vi "Filter and Connect Device.vi"() -> ()   [LabVIEW 2022 SP3]
doc: "In this example we will search through available devices to find the first one that has its \nmanufacturer set to 'openDAQ'.Then connect the device into our component tree as a child device."
uses:
  Public/Classes/IInstance/IInstance.lvclass
  Public/Classes/IInstanceBuilder/IInstanceBuilder.lvclass
  Public/Classes/IDevice/IDevice.lvclass
  Public/Classes/IDeviceInfo/IDeviceInfo.lvclass
panel:
  out "connected devices":string[](array[string])
  out "error out":errorcluster
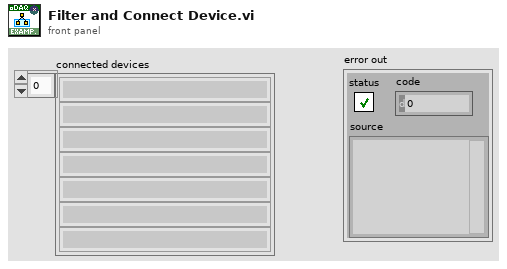
[diagram p1: front panel]
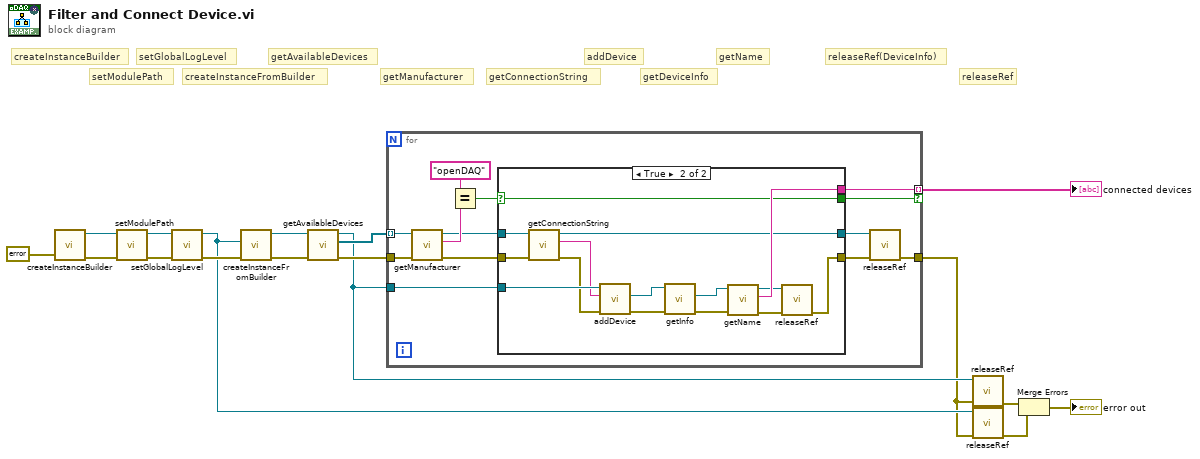
[diagram p0: block diagram]
diagram:
  # "getName"
  # "getDeviceInfo"
  # "addDevice"
  # "getConnectionString"
  # "createInstanceFromBuilder"
  # "releaseRef(DeviceInfo)"
  # "getManufacturer"
  # "releaseRef"
  # "getAvailableDevices"
  # "setGlobalLogLevel"
  # "setModulePath"
  # "createInstanceBuilder"
  n1 = call "createInstanceBuilder.vi"("error in (no error)"=errorcluster {"status"=FALSE, "code"=0, "source"=""}) -> ("error out"=w16:errorcluster, "IInstanceBuilder out"=w15:refnum<class "IInstanceBuilder.lvclass">)  [unwired: 9 in]
  n2 = call "setModulePath.vi"("error in (no error)"=w16, "IInstanceBuilder in"=w15) -> ("error out"=w14:errorcluster, "IInstanceBuilder out"=w13:refnum<class "IInstanceBuilder.lvclass">)  [unwired: 8 in]
  n3 = call "setGlobalLogLevel.vi"("error in (no error)"=w14, "IInstanceBuilder in"=w13) -> ("error out"=w11:errorcluster, "IInstanceBuilder out"=w7:refnum<class "IInstanceBuilder.lvclass">)  [unwired: 8 in]
  n4 = call "createInstanceFromBuilder.vi"("error in (no error)"=w11, "IInstanceBuilder in"=w7) -> ("error out"=w10:errorcluster, "IInstance out"=w9:refnum<class "IInstance.lvclass">)  [unwired: 8 in]
  n5 = call "getAvailableDevices.vi"("error in (no error)"=w10, "IDevice in"=w9) -> ("error out"=w17:errorcluster, "availableDeviceInfo out"=w8:refnum<class "IDeviceInfo.lvclass">[], "IDevice out"=w3:refnum<class "IInstance.lvclass">)  [unwired: 7 in]
  n6 = for {
    tunnel: w8 -> [w28] mode=indexing
    tunnel: w17 -> [w27]
    tunnel: [w29] -> w1
    tunnel: w3 -> [w20]
    tunnel: [w19] -> w2 mode=indexing if=w18
    n7 = call "getManufacturer.vi"("error in (no error)"=w27, "IDeviceInfo in"=w28) -> ("error out"=w30:errorcluster, "Manufacturer out"=w26:string, "IDeviceInfo out"=w23:refnum<class "IDeviceInfo.lvclass">)  [unwired: 7 in]
    n8 = Equal?(x=w26, y="openDAQ") -> (x = y?=w24:bool)
    n9 = case shown="True" w24 {
      selector: w24 -> [w31 w34]
      tunnel: w23 -> [w33 w47]
      tunnel: w30 -> [w32 w46]
      tunnel: [w33 w43] -> w22
      tunnel: [w32 w35] -> w21
      tunnel: w20 -> [_ w45]
      tunnel: [_ w48] -> w19
      tunnel: [w31 w34] -> w18
      frame False {
      }
      frame True {
        n10 = call "getConnectionString.vi"("error in (no error)"=w46, "IDeviceInfo in"=w47) -> ("error out"=w44:errorcluster, "ConntectionString out"=w42:string, "IDeviceInfo out"=w43:refnum<class "IDeviceInfo.lvclass">)  [unwired: 7 in]
        n11 = call "addDevice.vi"("error in (no error)"=w44, "ConnectionString in"=w42, "IDevice in"=w45) -> ("error out"=w39:errorcluster, "ConnectedDevice out"=w40:refnum<class "IDevice.lvclass">)  [unwired: 6 in, 1 out]
        n12 = call "getInfo.vi"("error in (no error)"=w39, "IDevice in"=w40) -> ("error out"=w38:errorcluster, "IDeviceInfo out"=w41:refnum<class "IDeviceInfo.lvclass">)  [unwired: 7 in, 1 out]
        n13 = call "getName.vi"("error in (no error)"=w38, "IDeviceInfo in"=w41) -> ("error out"=w36:errorcluster, "Name out"=w48:string, "IDeviceInfo out"=w37:refnum<class "IDeviceInfo.lvclass">)  [unwired: 7 in]
        n14 = call-dynamic "releaseRef.vi"("error in (no error)"=w36, "IBaseObject in"=w37) -> ("error out"=w35:errorcluster)  [unwired: 9 in]
      }
    }
    n15 = call-dynamic "releaseRef.vi"("error in (no error)"=w21, "IBaseObject in"=w22) -> ("error out"=w29:errorcluster)  [unwired: 9 in]
  }
  "connected devices" <- w2
  n16 = call-dynamic "releaseRef.vi"("error in (no error)"=w1, "IBaseObject in"=w3) -> ("error out"=w6:errorcluster)  [unwired: 9 in]
  n17 = call-dynamic "releaseRef.vi"("error in (no error)"=w1, "IBaseObject in"=w7) -> ("error out"=w5:errorcluster)  [unwired: 9 in]
  n18 = Merge Errors(w6, w5) -> (→"error out":errorcluster)
